vi "sCMOS_image_Contrast.vi"(3 "error in":errorcluster, 4 "Image Dst":T2, 5 "Image contrast":cluster{i32, i32}(slide) scale=0.0..16000.0, 6 "New Image":T2) -> (0 "error out":errorcluster, 1 "Image Dst Out":T2, 2 "Global Report":T1 {"Mean Value" format="%.2f"; "%" format="%.2f"; "Area (calibrated)" format="%.2f"; "Maximal Value" format="%.2f"; "Minimal Value" format="%.2f"; "Standard Variation" format="%.2f"})   [LabVIEW 2015]
uses:
  <vilib>/vision/Image Controls.llb/IMAQ Image.ctl
  <vilib>/vision/NI_Vision_Development_Module.lvlib
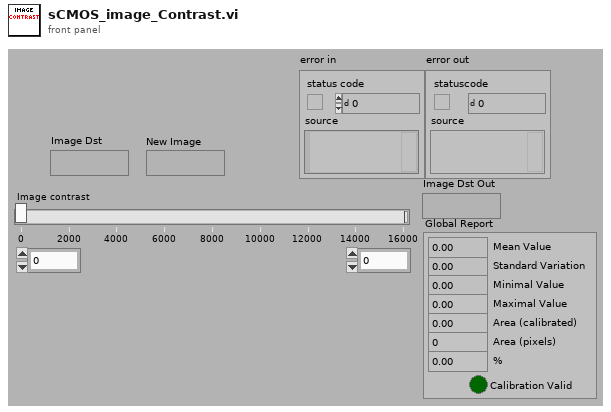
[diagram p1: front panel]
types:
  T1 = cluster{"Mean Value":sgl, "Standard Variation":sgl, "Minimal Value":sgl, "Maximal Value":sgl, "Area (calibrated)":sgl, "Area (pixels)":u32, "%":sgl, "Calibration Valid":bool}
  T2 = typedef "IMAQ Image.ctl" = refnum<image>
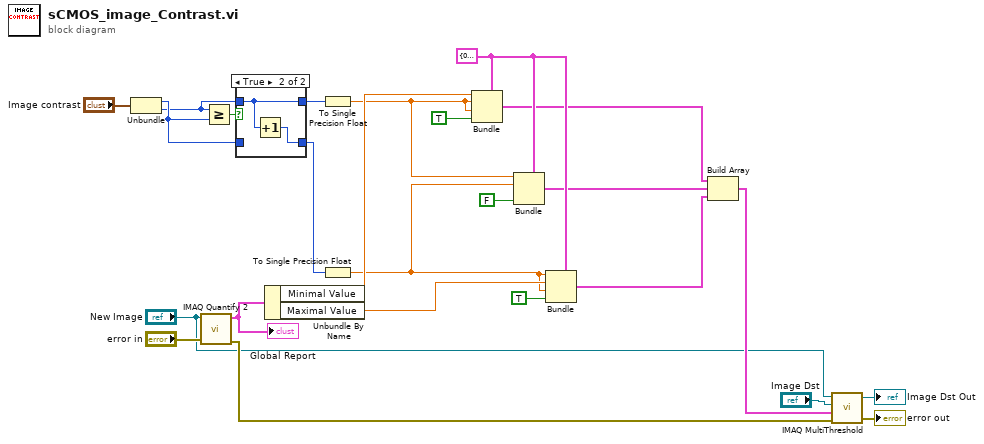
[diagram p0: block diagram]
diagram:
  w22 = cluster{sgl, sgl, sgl, bool} {0.0, 0.0, 0.0, TRUE}
  n1 = Unbundle("Image contrast") -> (w3:i32, w2:i32)
  n2 = call "IMAQ Quantify 2"("error in (no error)"="error in", "Image"="New Image") -> ("error out"=w12:errorcluster, "Global Report"=w11:T1)  [unwired: 7 in, 1 out]
  "Global Report" <- w11
  n3 = Greater Or Equal?(x=w2, y=w3) -> (x >= y?=w21:bool)
  n4 = case shown="True" w21 {
    tunnel: w2 -> [w27 w29]
    tunnel: w3 -> [w26 _]
    tunnel: [w27 w29] -> w20
    tunnel: [w26 w28] -> w19
    frame False {
    }
    frame True {
      n5 = Increment(x=w29) -> (x+1=w28:i32)
    }
  }
  n6 = Unbundle By Name(w11) -> ("Minimal Value"=w10:sgl, "Maximal Value"=w9:sgl)
  n7 = To Single Precision Float(number=w20) -> (single precision float=w8:sgl)
  n8 = To Single Precision Float(number=w19) -> (single precision float=w7:sgl)
  n9 = Bundle(cluster=w22, w10, w8, w8, TRUE) -> (w18:cluster{sgl, sgl, sgl, bool})
  n10 = Bundle(cluster=w22, w8, w7, FALSE) -> (w17:cluster{sgl, sgl, sgl, bool})  [unwired: 1 in]
  n11 = Bundle(cluster=w22, w7, w9, w7, TRUE) -> (w16:cluster{sgl, sgl, sgl, bool})
  n12 = Build Array(w18, w17, w16) -> (w15:cluster{sgl, sgl, sgl, bool}[])
  n13 = call "IMAQ MultiThreshold"("error in (no error)"=w12, "Threshold Data"=w15, "Image Dst"="Image Dst", "Image Src"="New Image") -> ("error out"=→"error out":errorcluster, "Image Dst Out"=→"Image Dst Out":T2)  [unwired: 1 in]
